vi "test Should Reset Call Count To Zero and Called To False.vi"(8 "error in (no error)":errorcluster, 11 "TestCase in":refnum<class "Reset Behaviour.lvclass">) -> (0 "error out":errorcluster, 3 "TestCase out":refnum<class "Reset Behaviour.lvclass">)   [LabVIEW 2013, in "Reset Behaviour.lvclass"]
uses:
  Reset Behaviour.lvclass
  Core Classes/LabSpy/LabSpy.lvclass
  Core Classes/LabSpy/Results/Been Called.vi
  <vilib>/addons/_JKI Toolkits/VI Tester/TestCase.llb/TestCase.lvclass
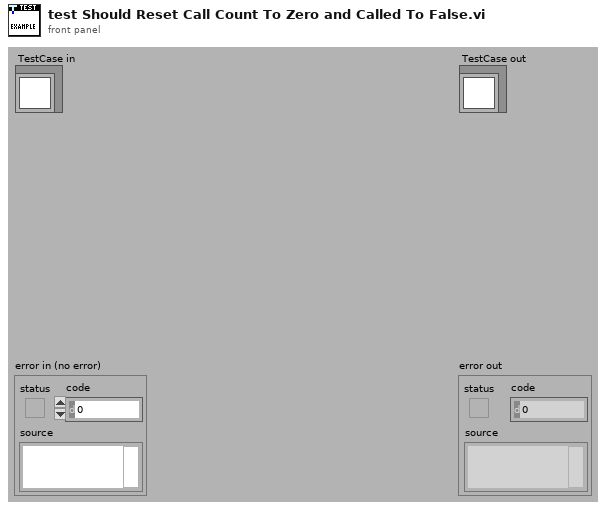
[diagram p1: front panel]
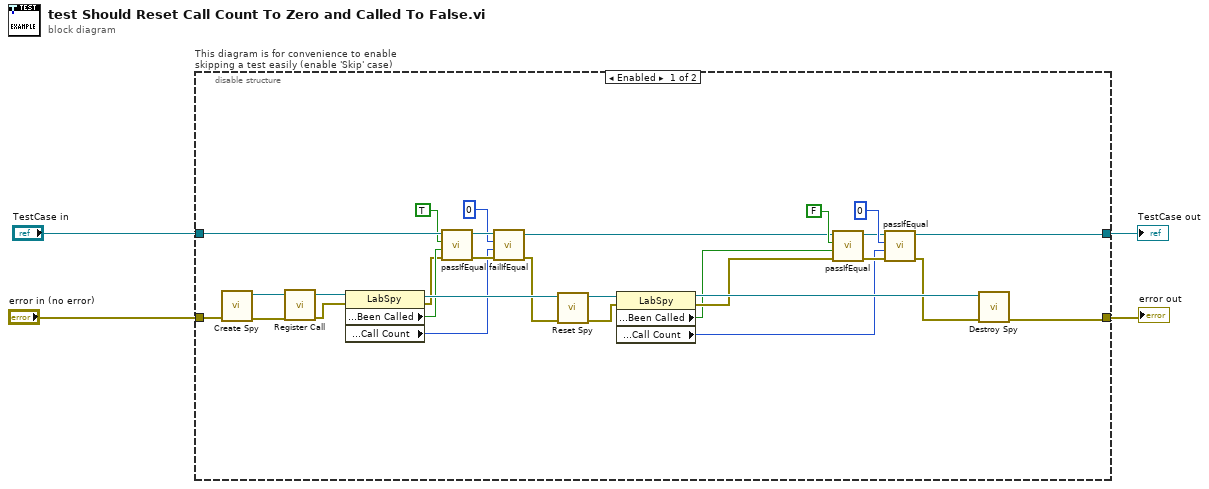
[diagram p0: block diagram]
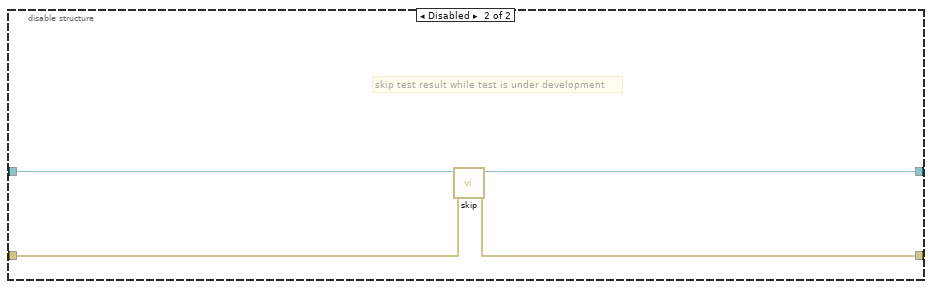
[diagram p2: hidden frame]
diagram:
  n1 = disable-structure "This diagram is for convenience to enable skipping a test easily (enable 'Skip' case)" shown="Enabled" {
    disable-tunnel: "TestCase in" -> [w24 w37]
    disable-tunnel: [w11 w35] -> w1
    disable-tunnel: [w8 w36] -> w3
    disable-tunnel: "error in (no error)" -> [w33 w34]
    frame Enabled {
      n2 = call "Create Spy.vi"("error in (no error)"=w33) -> ("error out"=w32:errorcluster, "LabSpy Out"=w31:refnum<data-value>)  [unwired: 9 in]
      n3 = call "Register Call.vi"("error in (no error)"=w32, "LabSpy"=w31) -> ("error out"=w30:errorcluster, "LabSpy Out"=w29:refnum<data-value>)  [unwired: 8 in]
      n4 = property class="LabSpy"(reference=w29, error in=w30) -> (reference out=w28:refnum<data-value>, error out=w20:errorcluster, "Call Monitoring:Been Called"=w21:bool, "Call Monitoring:Call Count"=w19:i32)
      n5 = call-dynamic "passIfEqual.vi"("error in (no error)"=w20, "y"=w21, "x"=TRUE ("Been Called"), "TestCase in"=w24) -> ("error out"=w23:errorcluster, "TestCase out"=w22:refnum<class "Reset Behaviour.lvclass">)  [unwired: 6 in]
      n6 = call-dynamic "failIfEqual.vi"("error in (no error)"=w23, "y"=w19, "x"=0 ("Call Count"), "TestCase in"=w22) -> ("error out"=w18:errorcluster, "TestCase out"=w12:refnum<class "Reset Behaviour.lvclass">)  [unwired: 6 in]
      n7 = call "Reset Spy.vi"("error in (no error)"=w18, "LabSpy"=w28) -> ("error out"=w26:errorcluster, "LabSpy Out"=w27:refnum<data-value>)  [unwired: 8 in]
      n8 = property class="LabSpy"(reference=w27, error in=w26) -> (reference out=w25:refnum<data-value>, error out=w10:errorcluster, "Call Monitoring:Been Called"=w6:bool, "Call Monitoring:Call Count"=w5:i32)
      n9 = call-dynamic "passIfEqual.vi"("error in (no error)"=w10, "y"=w6, "x"=FALSE ("Been Called"), "TestCase in"=w12) -> ("error out"=w7:errorcluster, "TestCase out"=w13:refnum<class "Reset Behaviour.lvclass">)  [unwired: 6 in]
      n10 = call-dynamic "passIfEqual.vi"("error in (no error)"=w7, "y"=w5, "x"=0 ("Call Count"), "TestCase in"=w13) -> ("error out"=w9:errorcluster, "TestCase out"=w11:refnum<class "Reset Behaviour.lvclass">)  [unwired: 6 in]
      n11 = call "Destroy Spy.vi"("error in (no error)"=w9, "LabSpy"=w25) -> ("error out"=w8:errorcluster)  [unwired: 9 in]
    }
    frame Disabled {
      # "skip test result while test is under development"
      n12 = call <vilib>:"skip.vi"("error in (no error)"=w34, "TestCase in"=w37) -> ("error out"=w36:errorcluster, "TestCase out"=w35:refnum<class "Reset Behaviour.lvclass">)  [unwired: 8 in]
    }
  }
  "error out" <- w3
  "TestCase out" <- w1
